vi "Initialize.vi"(8 "error in":errorcluster) -> (0 "error out":errorcluster, 3 "srp":T1)   [LabVIEW 2016, in "SRP.lvlib"]
uses:
  <vilib>/addons/InsightCM/SRP/SRP.lvlib
  <vilib>/addons/InsightCM/SRP/controls/DVR_data.ctl
  <vilib>/addons/InsightCM/SRP/controls/data.ctl
  <vilib>/addons/InsightCM/SRP/libraries/win32Urelease/brsrp.dll
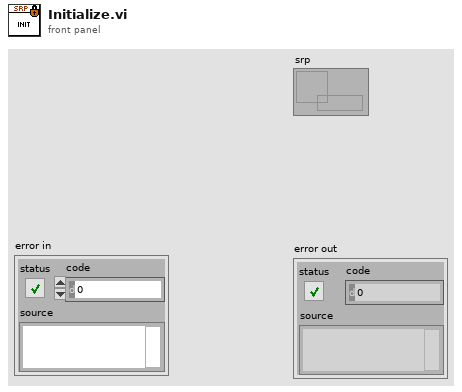
[diagram p1: front panel]
types:
  T1 = typedef "SRP.lvlib/DVR_data.ctl" = refnum<data-value>
  T2 = typedef "SRP.lvlib/data.ctl" = cluster{"SessionKey":u8[], "ClientHash":u8[], "PublicKeyA":u8[], "PrivateKeyA":u8[]}
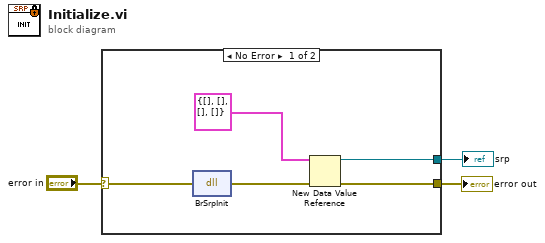
[diagram p0: block diagram]
diagram:
  n1 = case shown="No Error" "error in" {
    selector: "error in" -> [w8 w9]
    tunnel: [w5 w9] -> w3
    tunnel: [w4 _] -> w1
    frame No Error {
      n2 = dll-call lib="C:/Program Files (x86)/National Instruments/LabVIEW 2016/vi.lib/addons/InsightCM/SRP/libraries/win32Urelease/brsrp.*" fn="BrSrpInit"(error in=w8) -> (error out=w6:errorcluster)  [unwired: 3 in, 1 out]
      n3 = New Data Value Reference(data value=T2 {"SessionKey"=[], "ClientHash"=[], "PublicKeyA"=[], "PrivateKeyA"=[]} ("SrpData"), error in=w6) -> (data value reference=w4:refnum<data-value>, error out=w5:errorcluster)
    }
    frame Error {
    }
  }
  "error out" <- w3
  "srp" <- w1
